vi "PROVA-CONTROL-HYSTERESIS.vi"() -> ()   [LabVIEW 2015]
uses:
  VIPM2.lvlib
panel:
  out "Waveform Chart":sgl(graph)
  in  "Slide":sgl(slide) min=-20 max=100 step=0.02 scale=-20.0..100.0
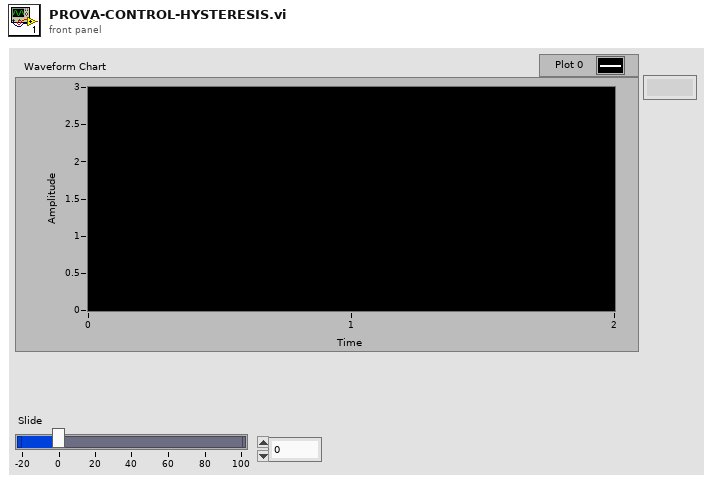
[diagram p1: front panel]
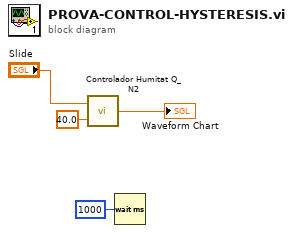
[diagram p0: block diagram]
diagram:
  n1 = call "Controlador Humitat Q_N2.vi"("Humidity setpoint (%RH)"=sgl 40.0, "Humidity (%RH)"="Slide") -> ("Q N2 setpoint (l/min)"=→"Waveform Chart":sgl)  [unwired: 1 in]
  n2 = Wait (ms)(milliseconds to wait=u32 1000) -> ()  [unwired: 1 out]
